vi "探头恢复出厂.vi"(7 "校准参数":u16(ring) caption="校准参数：" items=["pH", "DO", "浊度", "电导率", "叶绿素a", "藻密度", "ORP", "DO2", "氯化物"], 8 "error in (no error)":errorcluster caption="错误输入（无错误）") -> (0 "error out":errorcluster caption="错误输出")   [LabVIEW 2016, in "斯坦道多参数.lvlib"]
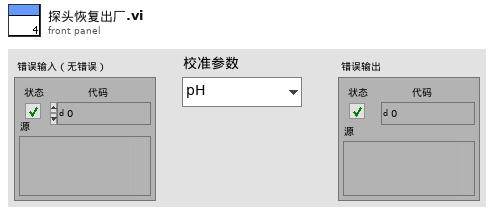
[diagram p1: front panel]
types:
  T1 = typedef "斯坦道多参数.lvlib/探头类型.ctl" = enum16{"禹山", "国弘", "纳清", "STD"}
  T2 = enum16{"null", "pH", "DO", "浊度", "电导率", "叶绿素a", "DO2"}
  T3 = enum16{"null", "pH", "DO", "浊度", "电导率", "叶绿素a", "DO2", "藻密度", "悬浮物"}
  T4 = enum16{"null", "pH", "DO", "浊度", "电导率", "叶绿素a", "DO2", "藻密度"}
  T5 = enum16{"NULL", "pH", "Cond", "DO", "Turb", "ORP"}
  T6 = enum16{"NULL", "pH", "Cond", "DO", "Turb", "ORP", "6", "7", "8", "9", "氯化物"}
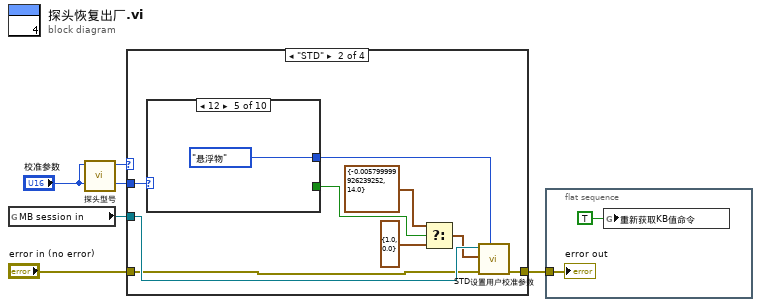
[diagram p0: block diagram]
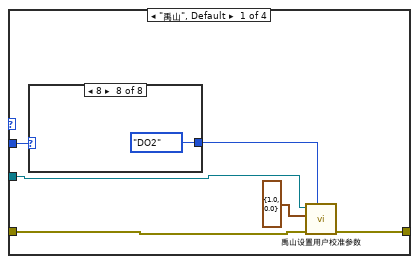
[diagram p2: hidden frame]
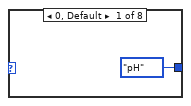
[diagram p3: hidden frame]
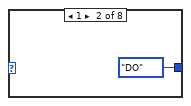
[diagram p4: hidden frame]
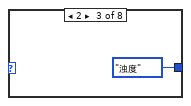
[diagram p5: hidden frame]
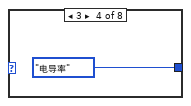
[diagram p6: hidden frame]
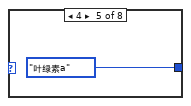
[diagram p7: hidden frame]
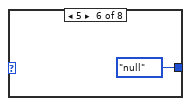
[diagram p8: hidden frame]
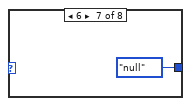
[diagram p9: hidden frame]
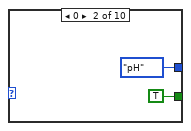
[diagram p11: hidden frame]
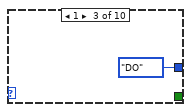
[diagram p12: hidden frame]
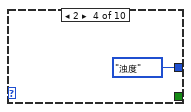
[diagram p13: hidden frame]
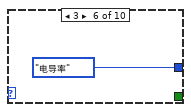
[diagram p14: hidden frame]
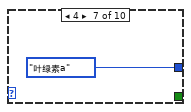
[diagram p15: hidden frame]
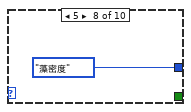
[diagram p16: hidden frame]
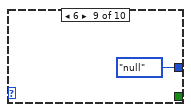
[diagram p17: hidden frame]
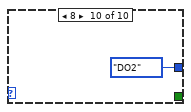
[diagram p18: hidden frame]
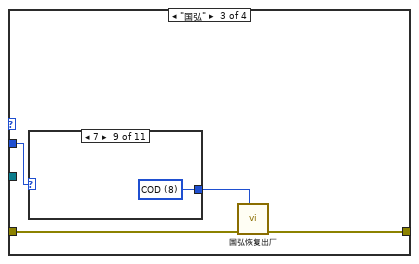
[diagram p19: hidden frame]
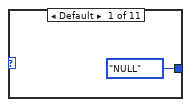
[diagram p20: hidden frame]
diagram:
  n1 = global read "多参数全局变量.vi" "MB session in"() -> (w1:refnum<class "MB_Master.lvclass">)
  n2 = call "探头型号.vi"("校准参数"="校准参数") -> ("探头型号"=w5:T1)  [unwired: 8 in, 2 out]
  n3 = case shown="\"STD\"" w5 {
    tunnel: "校准参数" -> [w11 w28 w42 _]
    tunnel: "error in (no error)" -> [w7 w25 w41 w54]
    tunnel: [w6 w24 w40 w54] -> w2
    tunnel: w1 -> [w8 w26 _ _]
    frame "禹山", Default {
      n4 = case shown="8" w11 {
        tunnel: [T2."pH" ("探头") T2."DO" ("探头") T2."浊度" ("探头") T2."电导率" ("探头") T2."叶绿素a" ("探头") T2."null" ("探头") T2."null" ("探头") T2."DO2" ("探头")] -> w9
        frame 0, Default {
        }
        frame 1 {
        }
        frame 2 {
        }
        frame 3 {
        }
        frame 4 {
        }
        frame 5 {
        }
        frame 6 {
        }
        frame 8 {
        }
      }
      n5 = call "禹山设置用户校准参数.vi"("探头"=w9, "error in (no error)"=w7, "用户校准参数"=cluster{"K":sgl, "B":sgl} {"K"=1.0, "B"=0.0}, "MB session in"=w8) -> ("error out"=w6:errorcluster)  [unwired: 6 in, 1 out]
    }
    frame "STD" {
      n6 = case shown="12" w28 {
        tunnel: [_ T2."pH" ("探头") T2."DO" ("探头") T2."浊度" ("探头") T3."悬浮物" ("探头") T2."电导率" ("探头") T2."叶绿素a" ("探头") T4."藻密度" ("探头") T2."null" ("探头") T2."DO2" ("探头")] -> w27
        tunnel: [_ TRUE _ _ _ _ _ _ _ _] -> w23
        frame Default {
        }
        frame 0 {
        }
        frame 1 {
        }
        frame 2 {
        }
        frame 12 {
        }
        frame 3 {
        }
        frame 4 {
        }
        frame 5 {
        }
        frame 6 {
        }
        frame 8 {
        }
      }
      n7 = Select(t=cluster{"K":sgl, "B":sgl} {"K"=-0.0058, "B"=14.0} ("用户校准参数"), s=w23, f=cluster{"K":sgl, "B":sgl} {"K"=1.0, "B"=0.0} ("用户校准参数")) -> (s? t:f=w20:cluster{"K":sgl, "B":sgl})
      n8 = call "STD设置用户校准参数.vi"("探头"=w27, "error in (no error)"=w25, "用户校准参数"=w20, "MB session in"=w26) -> ("error out"=w24:errorcluster)  [unwired: 6 in, 1 out]
    }
    frame "国弘" {
      n9 = case shown="7" w42 {
        tunnel: [T5."NULL" ("探头") T5."pH" ("探头") T5."DO" ("探头") T5."Turb" ("探头") T5."Cond" ("探头") T5."NULL" ("探头") T5."NULL" ("探头") T5."ORP" ("探头") w51 T6."氯化物" ("探头") 17] -> w39
        frame Default {
        }
        frame 0 {
        }
        frame 1 {
        }
        frame 2 {
        }
        frame 3 {
        }
        frame 4 {
        }
        frame 5 {
        }
        frame 6 {
        }
        frame 7 {
          w51 = u16 8 items=["NULL", "pH", "Cond", "DO", "Turb", "ORP", "6", "7", "COD", "9", "氯化物"] ("探头")
        }
        frame 9 {
        }
        frame 11 {
          # "水中油"
        }
      }
      n10 = call "国弘恢复出厂.vi"("探头"=w39, "error in (no error)"=w41) -> ("error out"=w40:errorcluster)  [unwired: 8 in, 1 out]
    }
    frame "纳清" {
    }
  }
  n11 = flat-sequence {
    tunnel: w2 -> [w56]
    frame #0 {
      n12 = global write "多参数全局变量.vi" "重新获取KB值命令"(TRUE ("重新获取KB值命令")) -> ()
      "error out" <- w56
    }
  }
